vi "SubVI_StopDecoder.vi"(8 "error in":errorcluster, 9 "decoder in":u64) -> (0 "error":errorcluster)   [LabVIEW 2021, in "DecodetoImage.lvlib"]
uses:
  DecodetoImage.lvlib
  niimaqdx.dll
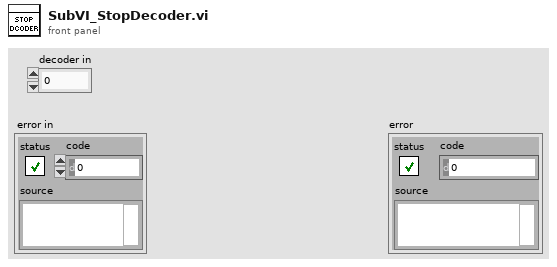
[diagram p1: front panel]
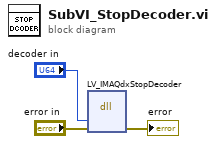
[diagram p0: block diagram]
diagram:
  n1 = dll-call lib="niimaqdx.dll" fn="LV_IMAQdxStopDecoder"("decoder"="decoder in", "error"="error in") -> ("error"=→"error":errorcluster)  [unwired: 3 in, 4 out]
